vi "Is Default Test.vi"(11 "Test in":refnum<class "Test.lvclass">) -> (2 "Is Default Test?":bool)   [LabVIEW 2018, in "Test.lvclass"]
doc: "For each data type, there should be one class which overrides this vi to define a default test. The default value is false. If no test is set to true, the first test is the default."
uses:
  Test.lvclass
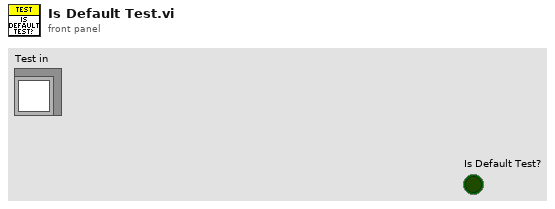
[diagram p1: front panel]
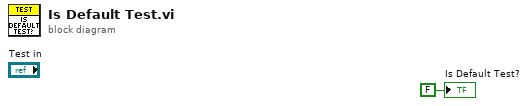
[diagram p0: block diagram]
diagram:
  "Is Default Test?" <- FALSE ("Is Default Test?")
